vi "Untitled 21.vi"(8 "error in":errorcluster) -> (0 "error out":errorcluster, 3 "task out":refnum<k21>)   [LabVIEW 2017]
uses:
  <vilib>/DAQmx/configure/timing.llb/DAQmx Timing (Sample Clock).vi
  <vilib>/DAQmx/create/channels.llb/DAQmx Create Channel (AO-Voltage-Basic).vi
  <resource>/objmgr/daqmx.rc
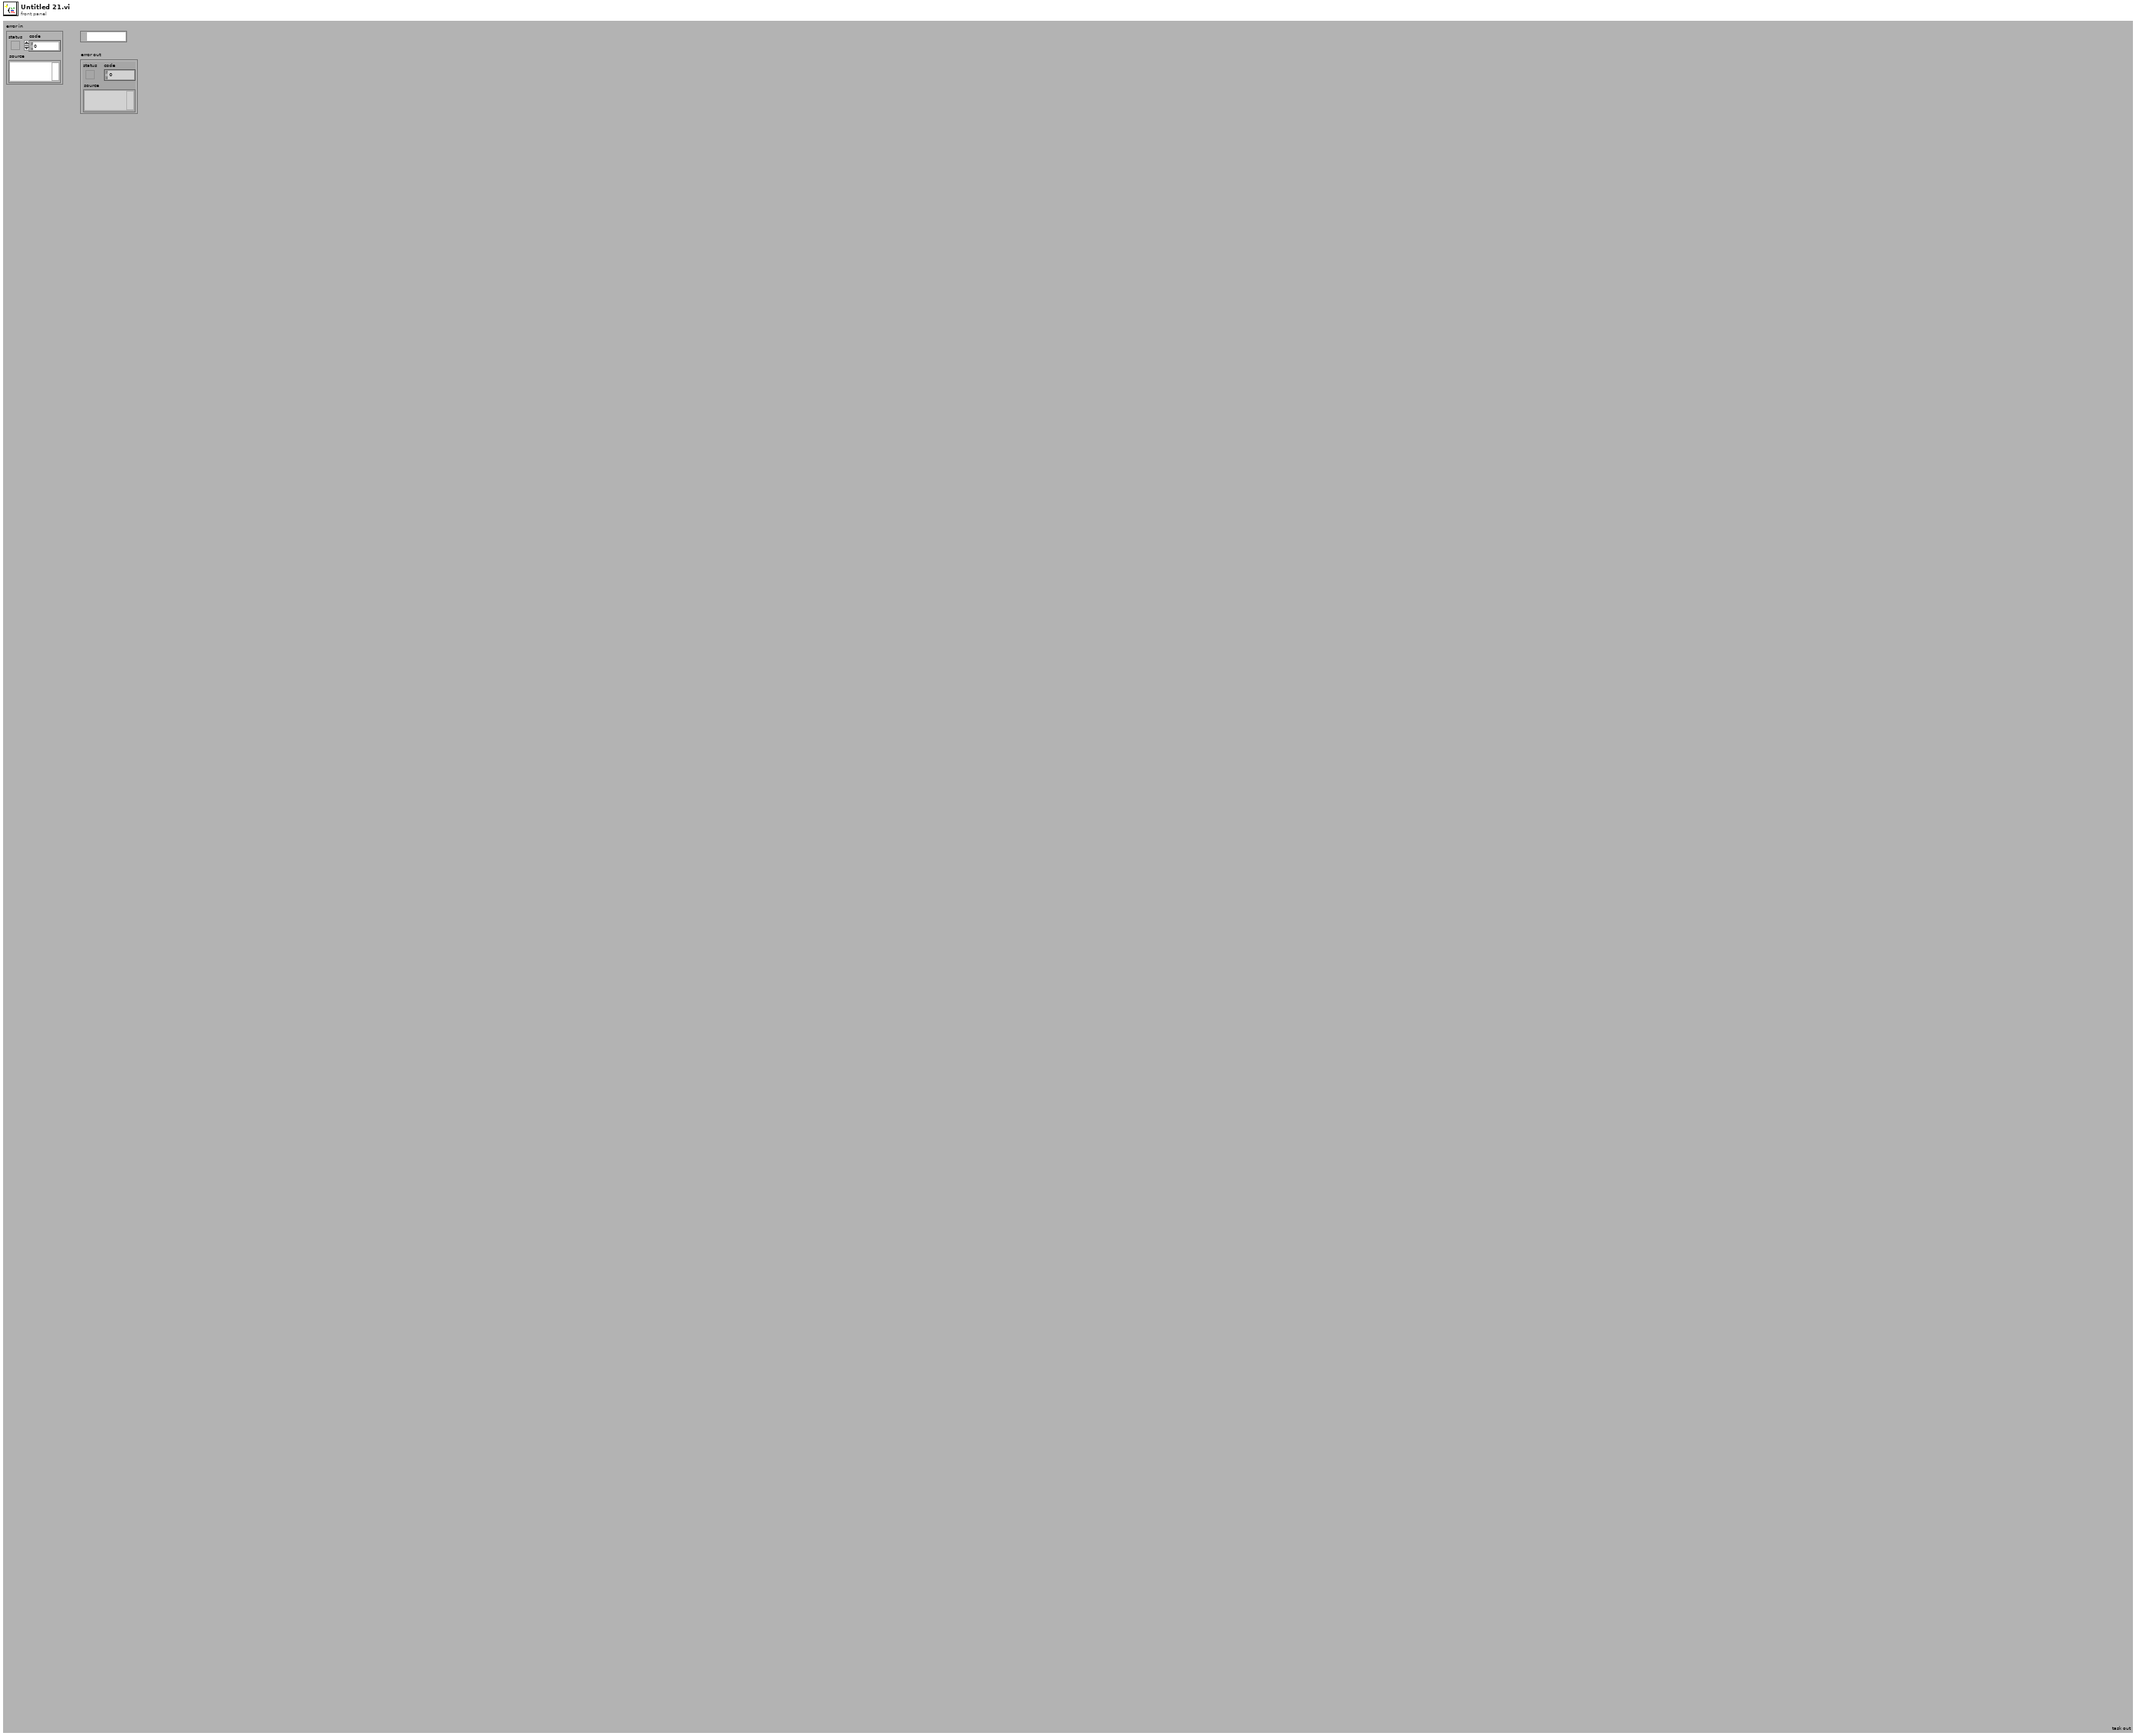
[diagram p1: front panel]
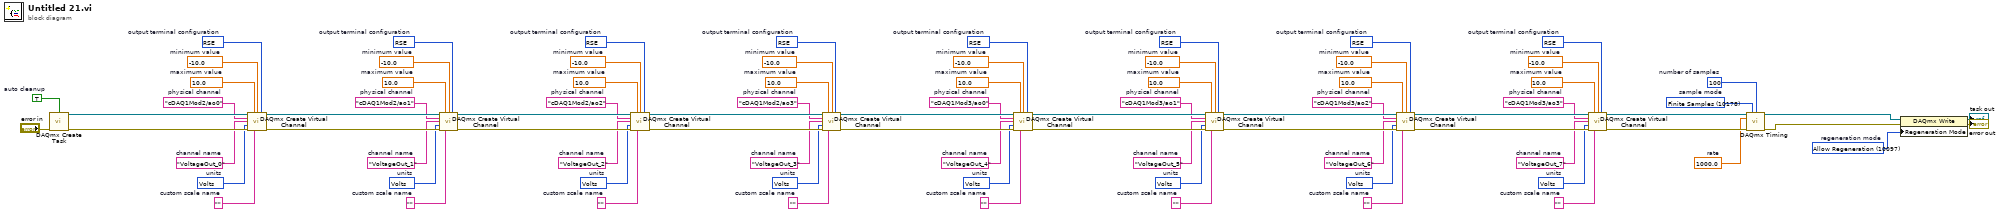
[diagram p0: block diagram]
diagram:
  w1 = 10097 items=["Allow Regeneration"=10097, "Do Not Allow Regeneration"=10158]  # regeneration mode
  w5 = 10178 items=["Finite Samples"=10178, "Continuous Samples"=10123, "Hardware Timed Single Point"=12522]  # sample mode
  w6 = 100  # number of samples
  w7 = 1000.0  # rate
  w10 = 10083 items=["Default"=-1, "RSE"=10083, "Differential"=10106, "Pseudodifferential"=12529]  # output terminal configuration
  w11 = 10348 items=["Volts"=10348, "From Custom Scale"=10065]  # units
  w12 = "VoltageOut_7"  # channel name
  w14 = ""  # custom scale name
  w15 = -10.0  # minimum value
  w16 = 10.0  # maximum value
  w17 = "cDAQ1Mod3/ao3"  # physical channel
  w19 = 10083 items=["Default"=-1, "RSE"=10083, "Differential"=10106, "Pseudodifferential"=12529]  # output terminal configuration
  w20 = 10348 items=["Volts"=10348, "From Custom Scale"=10065]  # units
  w21 = "VoltageOut_6"  # channel name
  w23 = ""  # custom scale name
  w24 = -10.0  # minimum value
  w25 = 10.0  # maximum value
  w26 = "cDAQ1Mod3/ao2"  # physical channel
  w28 = 10083 items=["Default"=-1, "RSE"=10083, "Differential"=10106, "Pseudodifferential"=12529]  # output terminal configuration
  w29 = 10348 items=["Volts"=10348, "From Custom Scale"=10065]  # units
  w30 = "VoltageOut_5"  # channel name
  w32 = ""  # custom scale name
  w33 = -10.0  # minimum value
  w34 = 10.0  # maximum value
  w35 = "cDAQ1Mod3/ao1"  # physical channel
  w37 = 10083 items=["Default"=-1, "RSE"=10083, "Differential"=10106, "Pseudodifferential"=12529]  # output terminal configuration
  w38 = 10348 items=["Volts"=10348, "From Custom Scale"=10065]  # units
  w39 = "VoltageOut_4"  # channel name
  w41 = ""  # custom scale name
  w42 = -10.0  # minimum value
  w43 = 10.0  # maximum value
  w44 = "cDAQ1Mod3/ao0"  # physical channel
  w46 = 10083 items=["Default"=-1, "RSE"=10083, "Differential"=10106, "Pseudodifferential"=12529]  # output terminal configuration
  w47 = 10348 items=["Volts"=10348, "From Custom Scale"=10065]  # units
  w48 = "VoltageOut_3"  # channel name
  w50 = ""  # custom scale name
  w51 = -10.0  # minimum value
  w52 = 10.0  # maximum value
  w53 = "cDAQ1Mod2/ao3"  # physical channel
  w55 = 10083 items=["Default"=-1, "RSE"=10083, "Differential"=10106, "Pseudodifferential"=12529]  # output terminal configuration
  w56 = 10348 items=["Volts"=10348, "From Custom Scale"=10065]  # units
  w57 = "VoltageOut_2"  # channel name
  w59 = ""  # custom scale name
  w60 = -10.0  # minimum value
  w61 = 10.0  # maximum value
  w62 = "cDAQ1Mod2/ao2"  # physical channel
  w64 = 10083 items=["Default"=-1, "RSE"=10083, "Differential"=10106, "Pseudodifferential"=12529]  # output terminal configuration
  w65 = 10348 items=["Volts"=10348, "From Custom Scale"=10065]  # units
  w66 = "VoltageOut_1"  # channel name
  w68 = ""  # custom scale name
  w69 = -10.0  # minimum value
  w70 = 10.0  # maximum value
  w71 = "cDAQ1Mod2/ao1"  # physical channel
  w73 = 10083 items=["Default"=-1, "RSE"=10083, "Differential"=10106, "Pseudodifferential"=12529]  # output terminal configuration
  w74 = 10348 items=["Volts"=10348, "From Custom Scale"=10065]  # units
  w75 = "VoltageOut_0"  # channel name
  w77 = ""  # custom scale name
  w78 = -10.0  # minimum value
  w79 = 10.0  # maximum value
  w80 = "cDAQ1Mod2/ao0"  # physical channel
  w82 = TRUE  # auto cleanup
  n1 = call <vilib>:"DAQmx Create Task.vi"("auto cleanup"=w82, "error in"="error in") -> ("task out"=w81:refnum<k21>, "error out"=w83:errorcluster)  [unwired: 12 in]
  n2 = call-poly <vilib>:"DAQmx Create Virtual Channel.vi"("task in"=w81, "maximum value"=w79, "minimum value"=w78, "output terminal configuration"=w73, "physical channels"=w80, "name to assign"=w75, "units"=w74, "error in"=w83, "custom scale name"=w77) -> ("task out"=w72:refnum<k21>, "error out"=w76:errorcluster)  [unwired: 5 in]
  n3 = call-poly <vilib>:"DAQmx Create Virtual Channel.vi"("task in"=w72, "maximum value"=w70, "minimum value"=w69, "output terminal configuration"=w64, "physical channels"=w71, "name to assign"=w66, "units"=w65, "error in"=w76, "custom scale name"=w68) -> ("task out"=w63:refnum<k21>, "error out"=w67:errorcluster)  [unwired: 5 in]
  n4 = call-poly <vilib>:"DAQmx Create Virtual Channel.vi"("task in"=w63, "maximum value"=w61, "minimum value"=w60, "output terminal configuration"=w55, "physical channels"=w62, "name to assign"=w57, "units"=w56, "error in"=w67, "custom scale name"=w59) -> ("task out"=w54:refnum<k21>, "error out"=w58:errorcluster)  [unwired: 5 in]
  n5 = call-poly <vilib>:"DAQmx Create Virtual Channel.vi"("task in"=w54, "maximum value"=w52, "minimum value"=w51, "output terminal configuration"=w46, "physical channels"=w53, "name to assign"=w48, "units"=w47, "error in"=w58, "custom scale name"=w50) -> ("task out"=w45:refnum<k21>, "error out"=w49:errorcluster)  [unwired: 5 in]
  n6 = call-poly <vilib>:"DAQmx Create Virtual Channel.vi"("task in"=w45, "maximum value"=w43, "minimum value"=w42, "output terminal configuration"=w37, "physical channels"=w44, "name to assign"=w39, "units"=w38, "error in"=w49, "custom scale name"=w41) -> ("task out"=w36:refnum<k21>, "error out"=w40:errorcluster)  [unwired: 5 in]
  n7 = call-poly <vilib>:"DAQmx Create Virtual Channel.vi"("task in"=w36, "maximum value"=w34, "minimum value"=w33, "output terminal configuration"=w28, "physical channels"=w35, "name to assign"=w30, "units"=w29, "error in"=w40, "custom scale name"=w32) -> ("task out"=w27:refnum<k21>, "error out"=w31:errorcluster)  [unwired: 5 in]
  n8 = call-poly <vilib>:"DAQmx Create Virtual Channel.vi"("task in"=w27, "maximum value"=w25, "minimum value"=w24, "output terminal configuration"=w19, "physical channels"=w26, "name to assign"=w21, "units"=w20, "error in"=w31, "custom scale name"=w23) -> ("task out"=w18:refnum<k21>, "error out"=w22:errorcluster)  [unwired: 5 in]
  n9 = call-poly <vilib>:"DAQmx Create Virtual Channel.vi"("task in"=w18, "maximum value"=w16, "minimum value"=w15, "output terminal configuration"=w10, "physical channels"=w17, "name to assign"=w12, "units"=w11, "error in"=w22, "custom scale name"=w14) -> ("task out"=w8:refnum<k21>, "error out"=w13:errorcluster)  [unwired: 5 in]
  n10 = call-poly <vilib>:"DAQmx Timing.vi"("task/channels in"=w8, "sample mode"=w5, "samples per channel"=w6, "rate"=w7, "error in"=w13) -> ("task out"=w4:refnum<k21>, "error out"=w9:errorcluster)  [unwired: 9 in]
  n11 = property class="DAQmx Write"(reference=w4, error in=w9, "Regeneration Mode"=w1) -> (reference out=→"task out":refnum<k21>, error out=→"error out":errorcluster)
